vi "Test 2.vi"   [LabVIEW 2024]
uses:
  Root Tester/Root Tester/Root Tester.lvclass
  C:/Program Files (x86)/National Instruments/LabVIEW 2024/vi.lib/ActorFramework/Actor/Actor.lvclass
  <vilib>/ActorFramework/Actor/Actor.lvclass
panel:
  # "ROOT TESTER LAUNCHER"
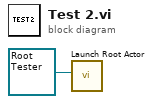
[diagram p0: block diagram]
diagram:
  n1 = call <vilib>:"Launch Root Actor.vi"("Actor"=refnum<class "Root Tester.lvclass"> refnum ("Root Tester.lvlib:Root Tester.lvclass")) -> ()  [unwired: 9 in, 2 out]
